vi "ASM.StatePostAction.vi"(8 "error in (no error)":errorcluster, 11 "ActorStateMachine in":refnum<class "ActorStateMachine.lvclass">) -> (0 "error out":errorcluster, 3 "ActorStateMachine out":refnum<class "ActorStateMachine.lvclass">)   [LabVIEW 2021, in "ActorStateMachine.lvlib" / "ActorStateMachine.lvclass"]
uses:
  ActorStateMachine.lvclass
  ActorStateMachine.lvclass/ActorStateMachine.ctl
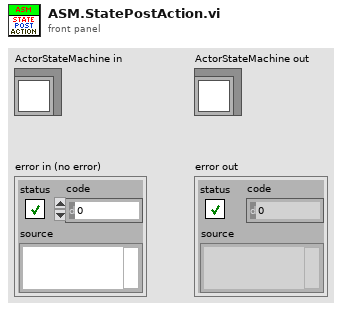
[diagram p1: front panel]
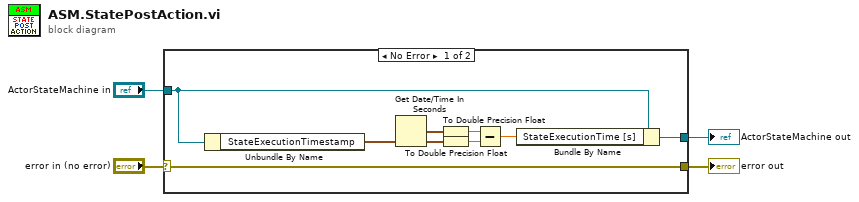
[diagram p0: block diagram]
diagram:
  n1 = case shown="No Error" "error in (no error)" {
    selector: "error in (no error)" -> [w6 w14]
    tunnel: [w6 w14] -> w3
    tunnel: [w5 w13] -> w1
    tunnel: "ActorStateMachine in" -> [w8 w13]
    frame No Error {
      n2 = Unbundle By Name(w8) -> ("StateExecutionTimestamp"=w7:timestamp)
      n3 = Get Date/Time In Seconds() -> (seconds since 1Jan1904=w9:timestamp)
      n4 = To Double Precision Float(number=w9) -> (double precision float=w11:dbl)
      n5 = To Double Precision Float(number=w7) -> (double precision float=w12:dbl)
      n6 = Subtract(x=w11, y=w12) -> (x-y=w10:dbl)
      n7 = Bundle By Name(cluster=w8, "StateExecutionTime [s]"=w10) -> (w5:refnum<class "ActorStateMachine.lvclass">)
    }
    frame Error {
    }
  }
  "error out" <- w3
  "ActorStateMachine out" <- w1
